vi "Set Instrument From Marker.vi"(8 "error in (no error)":errorcluster, 9 "Instrument Setting (0: Center Frequency)":i32(ring) items=["Center Frequency", "Center Frequency Step", "Start Frequency", "Stop Frequency", "Delta Span", "Delta Center Frequency", "Reference Level"], 10 "Active Marker (1: Marker1)":i32(ring)=1 items=["Marker1"=1, "Marker2"=2, "Marker3"=3, "Marker4"=4, "Marker5"=5, "Marker6"=6, "Marker7"=7, "Marker8"=8, "Marker9"=9, "Marker10"=10, "Marker11"=11, "Marker12"=12], 11 "VISA resource name":refnum<visa-resource-name>) -> (0 "error out":errorcluster, 3 "VISA resource name out":refnum<visa-resource-name>)   [LabVIEW 2018, in "Agilent MXA Series.lvlib"]
doc: "Sets the reference level or center frequency to the value of the selected marker.\n\n<B>Note:</B>\nYou can use this VI only under Swept SA measurement type."
uses:
  Agilent MXA Series.lvlib
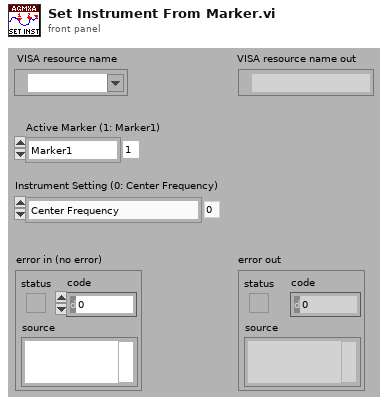
[diagram p1: front panel]
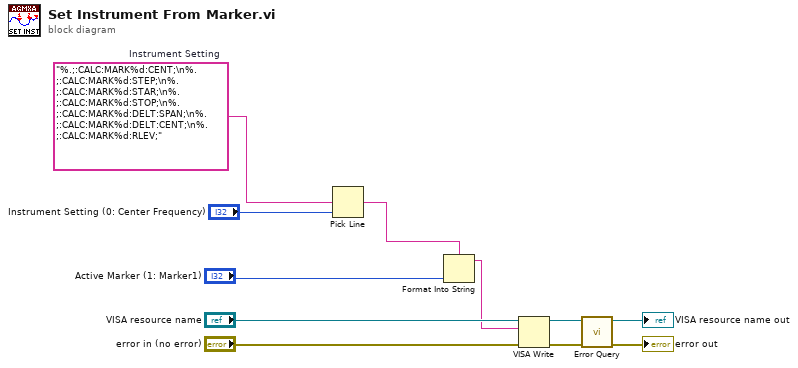
[diagram p0: block diagram]
diagram:
  w3 = "%.;:CALC:MARK%d:CENT;\n%.;:CALC:MARK%d:STEP;\n%.;:CALC:MARK%d:STAR;\n%.;:CALC:MARK%d:STOP;\n%.;:CALC:MARK%d:DELT:SPAN;\n%.;:CALC:MARK%d:DELT:CENT;\n%.;:CALC:MARK%d:RLEV;"  # Instrument Setting
  n1 = Pick Line(multi-line string=w3, line index="Instrument Setting (0: Center Frequency)") -> (output string=w2:string)  [unwired: 1 in]
  n2 = Format Into String(format string=w2, "Active Marker (1: Marker1)") -> (resulting string=w1:string)  [unwired: 2 in, 1 out]
  n3 = VISA Write(VISA resource name="VISA resource name", write buffer=w1, error in (no error)="error in (no error)") -> (VISA resource name out=w8:refnum<visa-resource-name>, error out=w6:errorcluster)  [unwired: 1 out]
  n4 = call "Error Query.vi"("error in (no error)"=w6, "VISA resource name"=w8) -> ("error out"=→"error out":errorcluster, "VISA resource name out"=→"VISA resource name out":refnum<visa-resource-name>)  [unwired: 6 in, 2 out]
